vi "AI Read & DO Digital write_기본코드.vi"() -> ()   [LabVIEW 2016]
doc: "Read one the value of one analog channel from a LINX device."
uses:
  <vilib>/MakerHub/LINX/Public/Peripherals/Analog/Analog Read 1 Chan.vi
  <vilib>/MakerHub/LINX/Public/Peripherals/Digital/Digital Write 1 Chan.vi
  <vilib>/MakerHub/LINX/Public/Peripherals/Analog/Analog Read N Chans.vi
  <vilib>/MakerHub/LINX/Public/Peripherals/Digital/Digital Write N Chans.vi
  <vilib>/MakerHub/LINX/Private/Local IO/LinxAnalogRead.vi
  <vilib>/MakerHub/LINX/Public/Utilities/Check Channel.vi
  <vilib>/MakerHub/LINX/Private/Local IO/LinxDigitalWrite.vi
  <vilib>/MakerHub/LINX/Public/Utilities/Open Serial.vi
  <vilib>/MakerHub/LINX/Private/Utilties/Generate Error.vi
  <vilib>/MakerHub/LINX/Public/Sensors/Motion/Servo/Servo Open One Channel.vi
  <vilib>/MakerHub/LINX/Public/Sensors/Motion/Servo/Servo Set Pulse Width One Channel.vi
  <vilib>/MakerHub/LINX/Public/Sensors/Motion/Servo/Servo Close One Channel.vi
  <vilib>/MakerHub/LINX/LMH-LINX.lvlib
  <vilib>/MakerHub/LINX/Public/Sensors/Motion/Servo/Servo.lvlib
panel:
  in  "Servo Channel 2":u8=2
  in  "T/F Control 2":bool
  in  "Digital Output Channel 2":u8=13
  in  "Servo Channel":u8=2
  in  "T/F Control":bool
  in  "Digital Output Channel":u8=13
  out "적외선AD(압력조건Off)":dbl(graph)
  in  "압력 룰베이스 INT 값":dbl
  out "적외선AD(압력조건On)":dbl(graph)
  out "Loop Rate (Hz)":u32
  in  "Stop Button":bool
  out "압력 AD":dbl(graph)
  in  "Serial Port":refnum<visa-resource-name>
  # "LINX Device Settings"
  # "적외선 센서(압력 조건 Fail)"
  # "압력 센서"
  # "적외선 센서(압력 조건 Pass)"
  # "Analog Read Example (Serial Interface)\n\nThis example demonstrates how to read analog input values from a LINX device connected to the host computer via Serial / USB.\n\nInstructions\n1. Select the COM Port associated with the LINX Device.\n2. Select the Analog Channel to read.\n3. Click the Run Arrow."
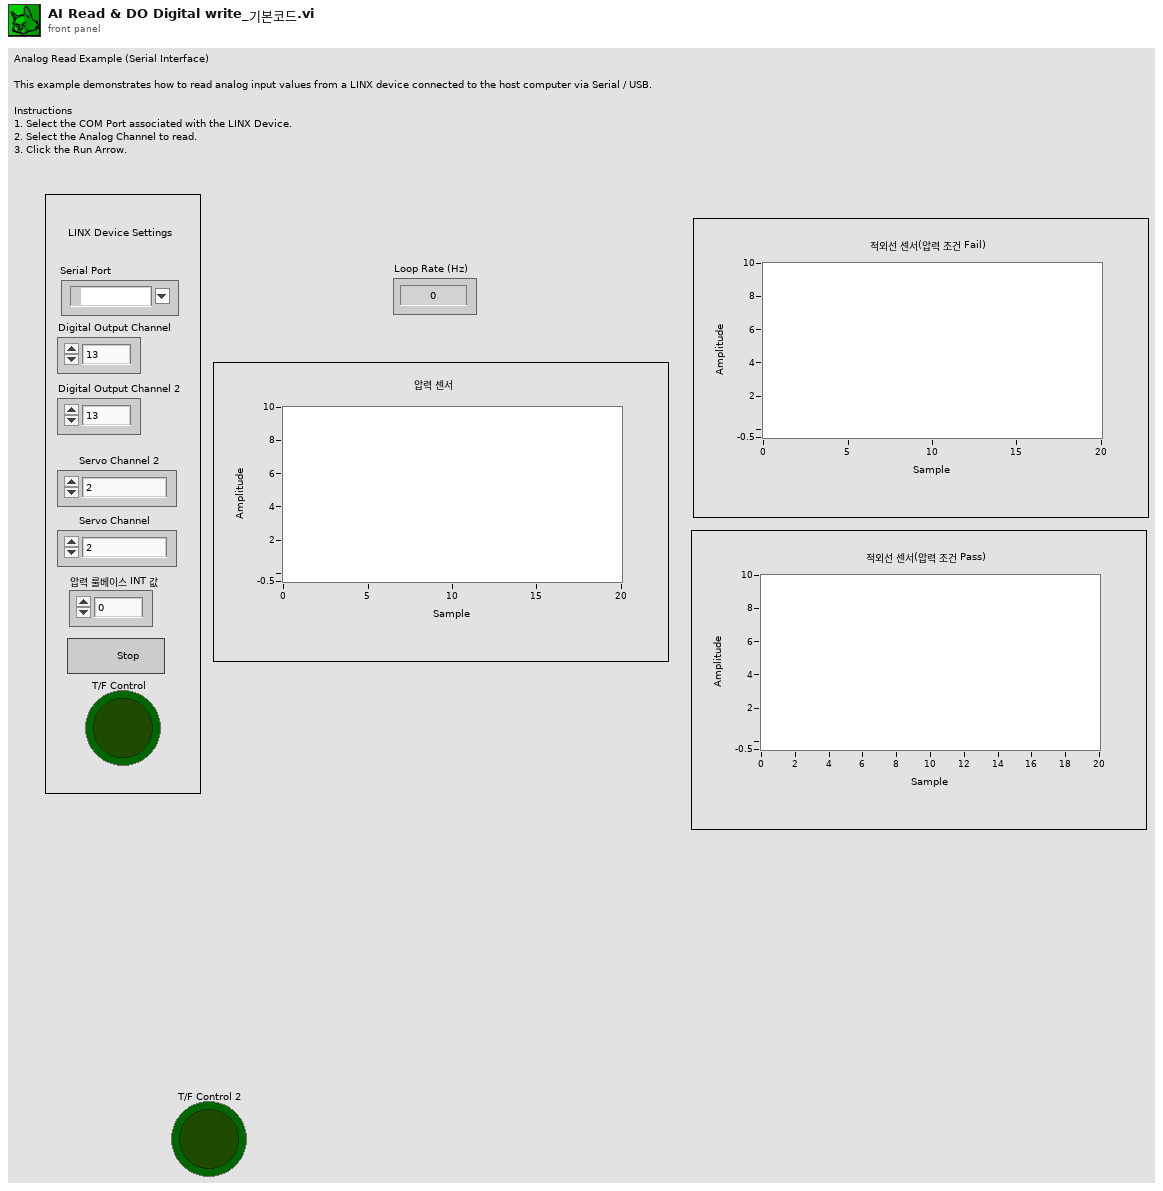
[diagram p1: front panel]
types:
  T1 = typedef "LMH-LINX.lvlib/LINX Ref.ctl" = cluster{"IO":T2, "Interface":T3, "LINX Device Config":T4}
  T2 = typedef "LMH-LINX.lvlib/Platform.ctl" = enum16{"Remote", "Local"}
  T3 = typedef "LMH-LINX.lvlib/Interface.ctl" = enum16{"Serial", "TCP"}
  T4 = typedef "LMH-LINX.lvlib/Device.lvlib/LINX Device Config.ctl" = cluster{"Interface":T3, "COM Port":refnum<visa-resource-name>, "TCP Configuration":T5, "Device Family":u8, "Device ID":u8, "Device Name":string, "TCP Ref":refnum<k5>, "Channels":T6}
  T5 = typedef "LMH-LINX.lvlib/Device.lvlib/TCP Config.ctl" = cluster{"IP Address":string, "Port":u16}
  T6 = typedef "LMH-LINX.lvlib/Channels.ctl" = cluster{"DI":u8[], "DO":u8[], "AI":u8[], "AO":u8[], "PWM":u8[], "QE":u8[], "UART":u8[], "I2C 2":u8[], "SPI":u8[], "CAN":u8[], "Servo":u8[], "AI Ref (V)":dbl, "AI Resolution (Bits)":u8, "AO Ref (V)":dbl, "AO Resolution (Bits)":u8}
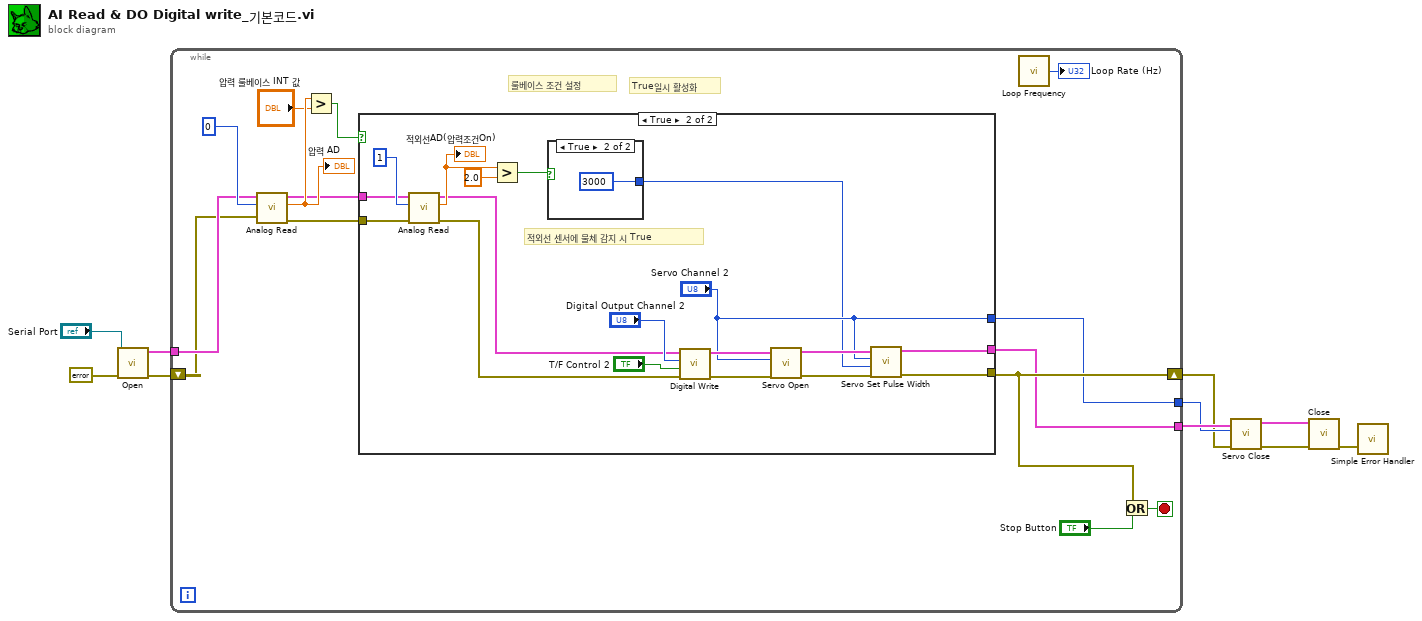
[diagram p0: block diagram]
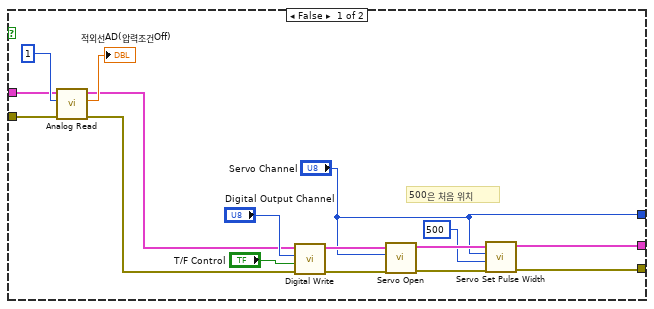
[diagram p2: hidden frame]
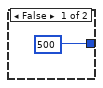
[diagram p3: hidden frame]
diagram:
  n1 = call-poly <vilib>:"Open.vi"("Error In"=errorcluster {"status"=FALSE, "code"=0, "source"=""}, "Serial Port"="Serial Port") -> ("Error Out"=w9:errorcluster, "LINX Resource"=w10:T1)  [unwired: 7 in, 1 out]
  n2 = while {
    tunnel: w10 -> [w17]
    shift-right: [w13] -> w1
    shift-left: w9 -> [w16]
    tunnel: [w11] -> w5
    tunnel: [w12] -> w2
    stop <- w24 stop-if-true
    # "True일시 활성화"
    # "룰베이스 조건 설정"
    n3 = call-poly <vilib>:"Analog Read.vi"("Error In"=w16, "Analog Channel"=u8 0 ("AI Channel"), "LINX Resource"=w17) -> ("Error Out"=w14:errorcluster, "Voltage"=w20:dbl, "LINX Resource"=w15:T1)  [unwired: 5 in, 1 out]
    "압력 AD" <- w20
    n4 = Greater?(x=w20, y="압력 룰베이스 INT 값") -> (0:w18:bool)
    n5 = case shown="True" w18 {
      tunnel: w15 -> [w38 w57]
      tunnel: w14 -> [w37 w56]
      tunnel: [w27 w43] -> w11
      tunnel: [w26 w45] -> w13
      tunnel: ["Servo Channel" "Servo Channel 2"] -> w12
      frame False {
        # "500은 처음 위치"
        n6 = call-poly <vilib>:"Analog Read.vi"("Error In"=w37, "Analog Channel"=u8 1, "LINX Resource"=w38) -> ("Error Out"=w29:errorcluster, "Voltage"=→"적외선AD(압력조건Off)":dbl, "LINX Resource"=w30:T1)  [unwired: 5 in, 1 out]
        n7 = call-poly <vilib>:"Digital Write.vi"("Error In"=w29, "Output Value"="T/F Control", "DO Channel"="Digital Output Channel", "LINX Resource"=w30) -> ("Error Out"=w34:errorcluster, "LINX Resource"=w35:T1)  [unwired: 6 in]
        n8 = call-poly <vilib>:"Servo Open.vi"("Error In"=w34, "Servo Channel"="Servo Channel", "LINX Resource"=w35) -> ("Error Out"=w32:errorcluster, "LINX Resource"=w33:T1)  [unwired: 7 in]
        n9 = call-poly <vilib>:"Servo Set Pulse Width.vi"("Error In"=w32, "Pulse Width (uS)"=u16 500, "Servo Channel"="Servo Channel", "LINX Resource"=w33) -> ("Error Out"=w26:errorcluster, "LINX Resource"=w27:T1)  [unwired: 6 in]
      }
      frame True {
        # "적외선 센서에 물체 감지 시 True"
        n10 = call-poly <vilib>:"Analog Read.vi"("Error In"=w56, "Analog Channel"=u8 1, "LINX Resource"=w57) -> ("Error Out"=w46:errorcluster, "Voltage"=w54:dbl, "LINX Resource"=w47:T1)  [unwired: 5 in, 1 out]
        "적외선AD(압력조건On)" <- w54
        n11 = Greater?(x=w54, y=2.0) -> (0:w42:bool)
        n12 = case shown="True" w42 {
          tunnel: [u16 500 ("Pulse Width (uS)") u16 3000 ("Pulse Width (uS)")] -> w41
          frame False {
          }
          frame True {
          }
        }
        n13 = call-poly <vilib>:"Digital Write.vi"("Error In"=w46, "Output Value"="T/F Control 2", "DO Channel"="Digital Output Channel 2", "LINX Resource"=w47) -> ("Error Out"=w51:errorcluster, "LINX Resource"=w52:T1)  [unwired: 6 in]
        n14 = call-poly <vilib>:"Servo Open.vi"("Error In"=w51, "Servo Channel"="Servo Channel 2", "LINX Resource"=w52) -> ("Error Out"=w49:errorcluster, "LINX Resource"=w50:T1)  [unwired: 7 in]
        n15 = call-poly <vilib>:"Servo Set Pulse Width.vi"("Error In"=w49, "Pulse Width (uS)"=w41, "Servo Channel"="Servo Channel 2", "LINX Resource"=w50) -> ("Error Out"=w45:errorcluster, "LINX Resource"=w43:T1)  [unwired: 6 in]
      }
    }
    n16 = call <vilib>:"Loop Frequency.vi"() -> ("Loop Rate (Hz)"=→"Loop Rate (Hz)":u32)
    n17 = Or(x=w13, y="Stop Button") -> (x .or. y?=w24:bool)
  }
  n18 = call-poly <vilib>:"Servo Close.vi"("Error In"=w1, "Servo Channel"=w2, "LINX Resource"=w5) -> ("Error Out"=w4:errorcluster, "LINX Resource"=w3:T1)  [unwired: 7 in]
  n19 = call <vilib>:"Close.vi"("Error In"=w4, "LINX Resource"=w3) -> ("Error Out"=w7:errorcluster)  [unwired: 9 in]
  n20 = call <vilib>:"Simple Error Handler.vi"("error in (no error)"=w7) -> ()  [unwired: 4 in, 5 out]
